vi "Main.vi"() -> ()   [LabVIEW 2017]
doc: "myRIO Rubik's Cube Solver App\n\nSmall test app turns and grips alls six servos. 3 grippers ands 3 turning servos.\n\n1) Configure PWM frequency, conversion from degrees to duty cycle\n2) Assign PWM channel to servo or gripper\n3) (Smart) Open PWM channel"
uses:
  <vilib>/myRIO/Instrument Drivers/Utilities/Utilities.lvlib
  <vilib>/ErrorRing/Error Ring.xnode
  ServoEnumControl.ctl
  ServoAbsAngleControl.ctl
panel:
  in  "Grip in":bool
  in  "Turn to":T1=-90 items=["-90°"=-90, "0°"=0, "+90°"=90]
  in  "Servo":T2
  out "Error":errorcluster
  in  "Stop":bool
  # "Test App: Turn and Grip Servos"
  # "Test two VI's\n\nServoSmartTurn.vi\nGripDoIt.vi"
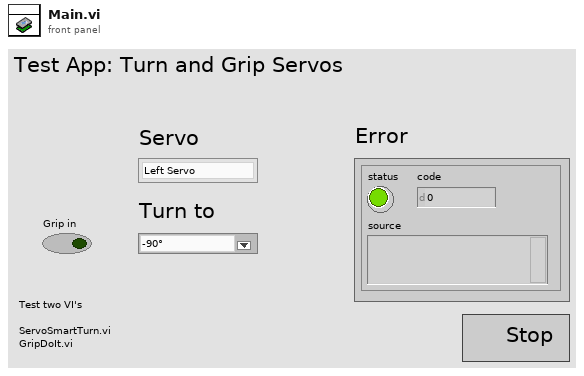
[diagram p1: front panel]
types:
  T1 = typedef "ServoAbsAngleControl.ctl" = i16
  T2 = typedef "ServoEnumControl.ctl" = enum16{"Left Servo", "Front Servo", "Right Servo"}
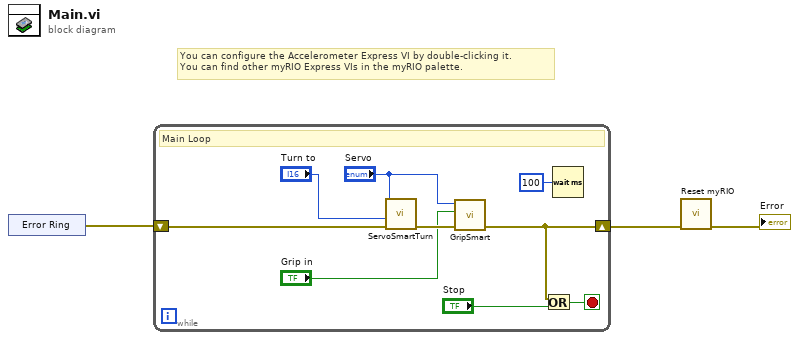
[diagram p0: block diagram]
diagram:
  # "You can configure the Accelerometer Express VI by double-clicking it.\nYou can find other myRIO Express VIs in the myRIO palette."
  n1 = xnode "Error Ring"() -> ("error out"=w2:errorcluster)
  n2 = while {
    shift-right: [w7] -> w1
    shift-left: w2 -> [w8]
    stop <- w11 stop-if-true
    # "Main Loop"
    n3 = call "ServoSmartTurn.vi"("error in"=w8, "Turn to (in)"="Turn to", "Servo"="Servo") -> ("error out"=w6:errorcluster)  [unwired: 7 in, 1 out]
    n4 = call "GripSmart.vi"("error in"=w6, "Turn to (in)"="Grip in", "Servo"="Servo") -> ("error out"=w7:errorcluster)  [unwired: 7 in, 1 out]
    n5 = Or(x=w7, y="Stop") -> (x .or. y?=w11:bool)
    n6 = Wait (ms)(milliseconds to wait=u32 100) -> ()  [unwired: 1 out]
  }
  n7 = call <vilib>:"Reset myRIO.vi"("error in (no error)"=w1) -> ("error out"=→"Error":errorcluster)  [unwired: 10 in]
